vi "WristNetwork.vi"(8 "error in (no error)":errorcluster) -> (0 "error out":errorcluster)   [LabVIEW 2023]
uses:
  WristGlobal.vi
  <vilib>/Rock Robotics/Network Tables/NT Write Number.vi
  <vilib>/Rock Robotics/Network Tables/NT Write Boolean.vi
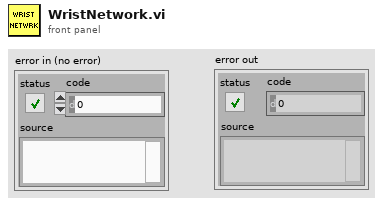
[diagram p1: front panel]
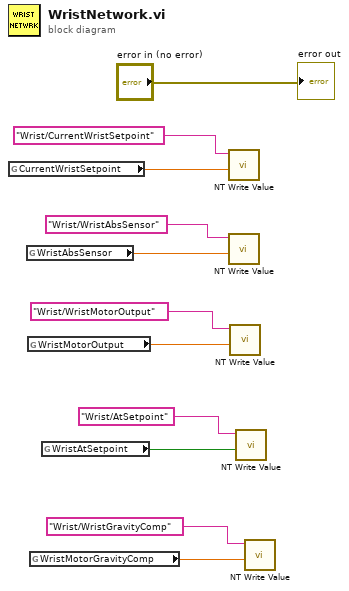
[diagram p0: block diagram]
diagram:
  n1 = global read "WristGlobal.vi" "CurrentWristSetpoint"() -> (w9:dbl)
  n2 = global read "WristGlobal.vi" "WristAbsSensor"() -> (w10:dbl)
  n3 = global read "WristGlobal.vi" "WristMotorOutput"() -> (w11:dbl)
  n4 = global read "WristGlobal.vi" "WristMotorGravityComp"() -> (w3:dbl)
  n5 = global read "WristGlobal.vi" "WristAtSetpoint"() -> (w5:bool)
  n6 = call-poly <vilib>:"NT Write Value.vi"("value"=w9, "name"="Wrist/CurrentWristSetpoint") -> ()  [unwired: 9 in, 1 out]
  n7 = call-poly <vilib>:"NT Write Value.vi"("value"=w10, "name"="Wrist/WristAbsSensor") -> ()  [unwired: 9 in, 1 out]
  n8 = call-poly <vilib>:"NT Write Value.vi"("value"=w11, "name"="Wrist/WristMotorOutput") -> ()  [unwired: 9 in, 1 out]
  n9 = call-poly <vilib>:"NT Write Value.vi"("value"=w5, "name"="Wrist/AtSetpoint") -> ()  [unwired: 9 in, 1 out]
  n10 = call-poly <vilib>:"NT Write Value.vi"("value"=w3, "name"="Wrist/WristGravityComp") -> ()  [unwired: 9 in, 1 out]
  "error out" <- "error in (no error)"
